vi "Reef Angle Adjustment.vi"(1 "Angle Align":bool=TRUE, 2 "April Tag ID":dbl, 3 "Robot Velocities":T2={"X Velocity"=0.17874253397302353, "Y Velocity"=3.0, "Rotational \nVelocity"=0.0}, 4 "PigeonIMUDevRef":T3={"DeviceStatus"={"status"=FALSE, "code"=0, "source"=""}, "Device Number"=21, "Type"=352321536, "Device ID"=352321557, "Handle"=23350768, "UsageFrame"=0, "Library Path"=path "libCTRE_PhoenixCCI.so"} {"Type" items=["CAN"=352321536, "TalonSRX"=33554432]}) -> (0 "Robot Velocties":T2={"X Velocity"=0.17874253397302353, "Y Velocity"=3.0, "Rotational \nVelocity"=0.0})   [LabVIEW 2023]
uses:
  <vilib>/Rock Robotics/WPI/ThirdParty/Phoenix-LabVIEW/Pigeon IMU/CTRE_PigeonIMU_DeviceRef.ctl
  <vilib>/Rock Robotics/WPI/ThirdParty/Phoenix-LabVIEW/Pigeon IMU/CTRE_PigeonIMU_ConnectionType.ctl
  swerve/Type Definitions/Data/Robot Velocities.ctl
  <vilib>/Rock Robotics/WPI/ThirdParty/Phoenix-LabVIEW/Pigeon IMU/CTRE_PigeonIMU_GetYPR.vi
  <vilib>/Rock Robotics/Network Tables/NT Read Numeric Array.vi
panel:
  in  "output range":cluster{"high":dbl, "low":dbl}={"high"=100.0, "low"=-100.0} {"low" format="%.2f"; "high" format="%.2f"}
  out "Waveform Chart":cluster{"output":dbl, "f":dbl}(graph)
  in  "PID gains":T1={"proportional gain (Kp)"=4.5, "integral time (Ki)"=0.0, "derivative time (Kd)"=0.0} {"derivative time (Kd)" format="%.3f"; "integral time (Ki)" format="%.3f"; "proportional gain (Kp)" format="%.3f"}
  in  "Angle Deadband":dbl=1.5
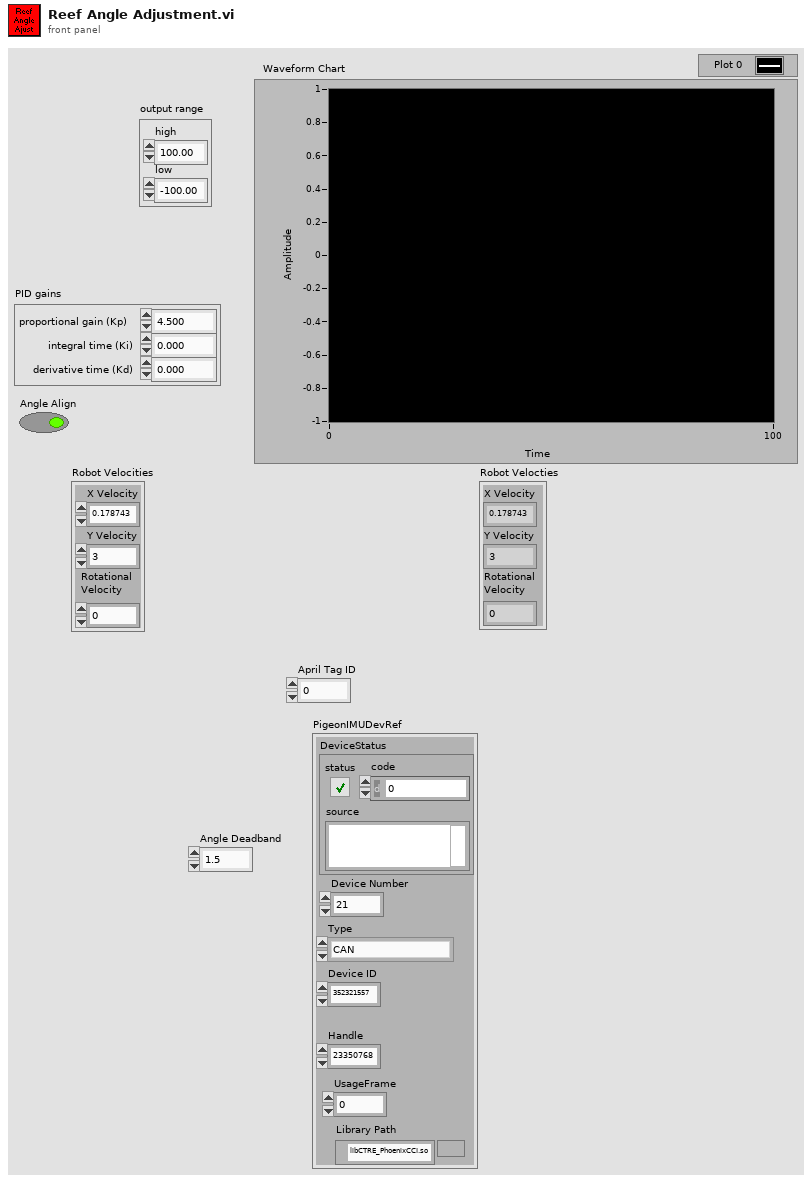
[diagram p1: front panel]
types:
  T1 = cluster{"proportional gain (Kp)":dbl, "integral time (Ki)":dbl, "derivative time (Kd)":dbl}
  T2 = typedef "Robot Velocities.ctl" = cluster{"X Velocity":dbl, "Y Velocity":dbl, "Rotational \nVelocity":dbl}
  T3 = typedef "CTRE_PigeonIMU_DeviceRef.ctl" = cluster{"DeviceStatus":errorcluster, "Device Number":u8, "Type":T4, "Device ID":u32, "Handle":u64, "UsageFrame":u32, "Library Path":path}
  T4 = typedef "CTRE_PigeonIMU_ConnectionType.ctl" = u32
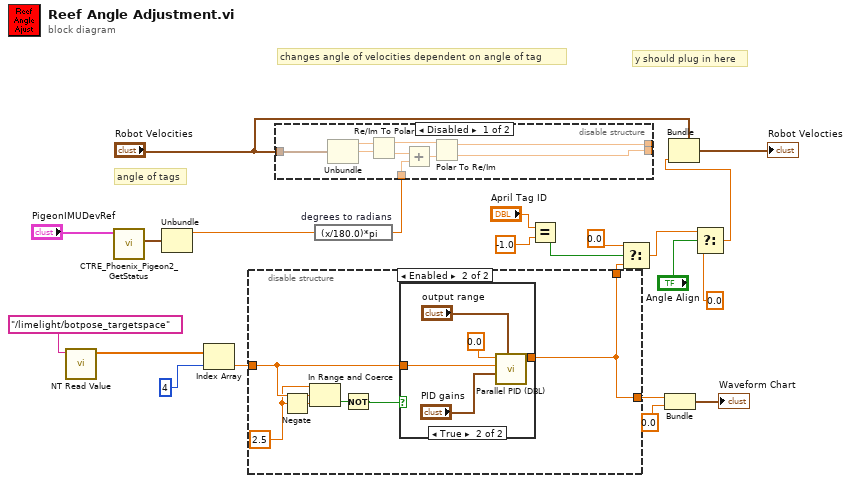
[diagram p0: block diagram]
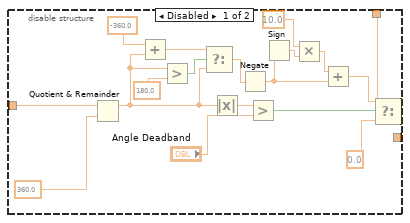
[diagram p2: hidden frame]
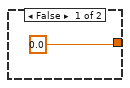
[diagram p3: hidden frame]
diagram:
  # "y should plug in here"
  # "changes angle of velocities dependent on angle of tag"
  # "angle of tags"
  n1 = call-poly <vilib>:"NT Read Value.vi"("name"="/limelight/botpose_targetspace") -> ("value"=w7:dbl[])  [unwired: 8 in, 2 out]
  n2 = call-poly <vilib>:"CTRE_Phoenix_Pigeon2_GetStatus.vi"("PigeonIMUDevRef"="PigeonIMUDevRef") -> ("Yaw Pitch Roll"=w21:cluster{"Yaw":dbl, "Pitch":dbl, "Roll":dbl})  [unwired: 8 in, 2 out]
  n3 = Unbundle(w21) -> ("Yaw"=w5:dbl)  [unwired: 2 out]
  n4 = Index Array(array=w7, index=4) -> (element=w6:dbl)
  n5 = disable-structure shown="Enabled" {
    disable-tunnel: [w24 w46] -> w18
    disable-tunnel: w6 -> [w23 w45]
    disable-tunnel: [_ w46] -> w3
    frame Disabled {
      n6 = Quotient & Remainder(x=w23, y=360.0) -> (x-y*floor(x/y)=w32:dbl)  [unwired: 1 out]
      n7 = Add(x=-360.0, y=w32) -> (x+y=w33:dbl)
      n8 = Greater?(x=w32, y=180.0) -> (0:w31:bool)
      n9 = Select(t=w33, s=w31, f=w32) -> (s? t:f=w35:dbl)
      n10 = Absolute Value(x=w32) -> (abs(x)=w36:dbl)
      n11 = Negate(x=w35) -> (-x=w26:dbl)
      n12 = Greater?(x=w36, y="Angle Deadband") -> (0:w39:bool)
      n13 = Sign(1:w26) -> (0:w27:dbl)
      n14 = Multiply(x=10.0, y=w27) -> (x*y=w28:dbl)
      n15 = Add(x=w28, y=w26) -> (x+y=w29:dbl)
      n16 = Select(t=w29, s=w39, f=0.0) -> (s? t:f=w24:dbl)
    }
    frame Enabled {
      w43 = 2.5 ("upper limit")
      n17 = Negate(x=w43) -> (-x=w42:dbl)
      n18 = In Range and Coerce(upper limit=w43, x=w45, lower limit=w42) -> (In Range?=w44:bool)  [unwired: 1 out]
      n19 = Not(x=w44) -> (.not. x?=w41:bool)
      n20 = case shown="True" w41 {
        tunnel: [0.0 ("output") w50] -> w46
        tunnel: w45 -> [_ w48]
        frame False {
        }
        frame True {
          n21 = call <vilib>:"Parallel PID (DBL).vi"("output range"="output range", "PID gains"="PID gains", "process variable"=w48, "setpoint"=0.0) -> ("output"=w50:dbl)  [unwired: 4 in, 3 out]
        }
      }
    }
  }
  n22 = expression code="(x/180.0)*pi" "degrees to radians"(w5) -> (w22:dbl)
  n23 = disable-structure shown="Disabled" {
    disable-tunnel: w22 -> [w57 _]
    disable-tunnel: [w56 _] -> _
    disable-tunnel: "Robot Velocities" -> [w55 _]
    disable-tunnel: [w53 _] -> _
    frame Disabled {
      n24 = Unbundle(w55) -> ("X Velocity"=w61:dbl, "Y Velocity"=w54:dbl)  [unwired: 1 out]
      n25 = Re/Im To Polar(2:w54, 3:w61) -> (0:w60:dbl, 1:w59:dbl)
      n26 = Add(x=w60, y=w57) -> (x+y=w58:dbl)
      n27 = Polar To Re/Im(2:w58, 3:w59) -> (0:w53:dbl, 1:w56:dbl)
    }
    frame Enabled {
    }
  }
  n28 = Equal?(x="April Tag ID", y=-1.0) -> (x = y?=w15:bool)
  n29 = Select(t=0.0, s=w15, f=w18) -> (s? t:f=w13:dbl)
  n30 = Bundle("output"=w3, "f"=0.0) -> (→"Waveform Chart":cluster{"output":dbl, "f":dbl})  [unwired: 1 in]
  n31 = Select(t=w13, s="Angle Align", f=0.0) -> (s? t:f=w12:dbl)
  n32 = Bundle(cluster="Robot Velocities", "Rotational \nVelocity"=w12) -> (→"Robot Velocties":T2)  [unwired: 2 in]
